vi "IEEE 754 Boolean_Array_to_SGL_LV2012_NI Verified.vi"(7 "array bool":bool[](array[boolean]), 10 "Tab Control":enum32{"SGL to Binary", "Binary to SGL"}(tab), 11 "Decimal Number":sgl=-101.101 format="%.12f") -> (3 "Decimal Number":sgl=-101.101 format="%.12f")   [LabVIEW 2015]
doc: "This VI shows how LabVIEW stores SGL floating-point numbers in memory in binary format. The 32-bit binary number is based on the following IEEE 754 format:\n\n1 bit for the SIGN\n8 bits for the EXPONENT\n23 bits for the MANTISSA\n\nThe formula for the conversion is the following:\n\nSGL = (-1)^SIGN * 1.MANTISSA * 2^(EXPONENT-127)\n\nYou can use this VI to convert SGL numbers to their binary storage equivalent, and vice versa."
panel:
  out "Decimal Exponent":sgl=6.0 format="%.2f"
  out "Decimal Mantissa":sgl=1.5797031 format="%.8f"
  out "Binary Mantissa":bool[](array[boolean])=[TRUE, FALSE, FALSE, TRUE, FALSE, TRUE, FALSE, FALSE, FALSE, TRUE, TRUE, FALSE, FALSE, TRUE, TRUE, TRUE, FALSE, TRUE, TRUE, FALSE, TRUE, TRUE, FALSE]
  out "Binary Exponent":bool[](array[boolean])=[TRUE, FALSE, FALSE, FALSE, FALSE, TRUE, FALSE, TRUE]
  out "Sign":bool=TRUE
  out "Sign":bool=TRUE
  out "Binary Exponent":bool[](array[boolean])=[TRUE, FALSE, FALSE, FALSE, FALSE, TRUE, FALSE, TRUE]
  out "Binary Mantissa":bool[](array[boolean])=[TRUE, FALSE, FALSE, TRUE, FALSE, TRUE, FALSE, FALSE, FALSE, TRUE, TRUE, FALSE, FALSE, TRUE, TRUE, TRUE, FALSE, TRUE, TRUE, FALSE, TRUE, TRUE, FALSE]
  out "Decimal Mantissa":sgl=1.5797031 format="%.8f"
  out "Decimal Exponent":i32=6
  # "Overview: This VI allows the conversion from and to IEEE 754 floating point\nRequirement: LabVIEW 2012 (or compatible)\nInstructions:\n1.  Choose a tab to convert from Binary to SGL or from SGL to binary\n2.  Enter your number in SGL or Binary\n3.  Run the VI"
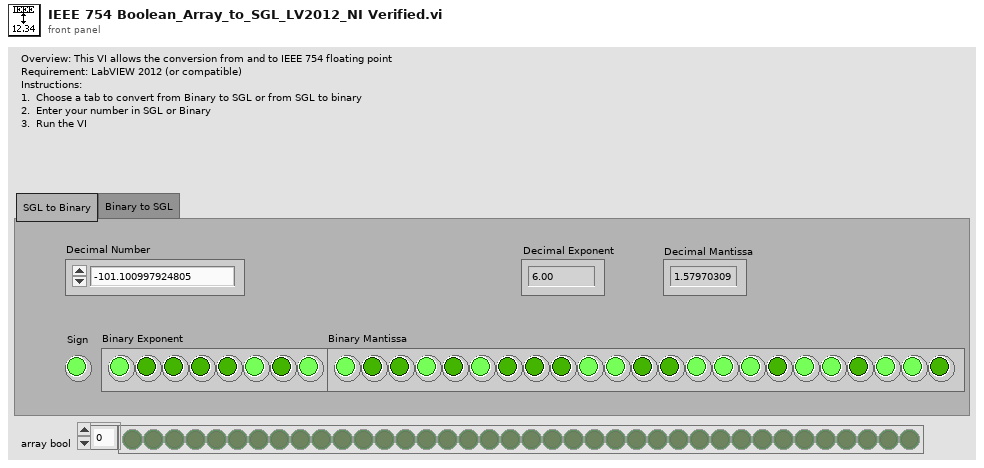
[diagram p1: front panel]
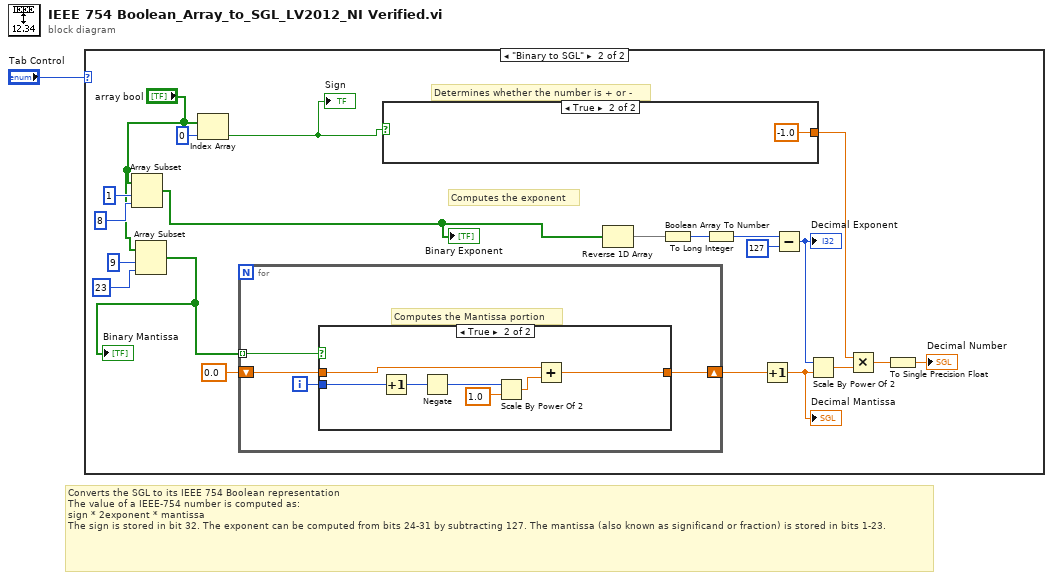
[diagram p0: block diagram]
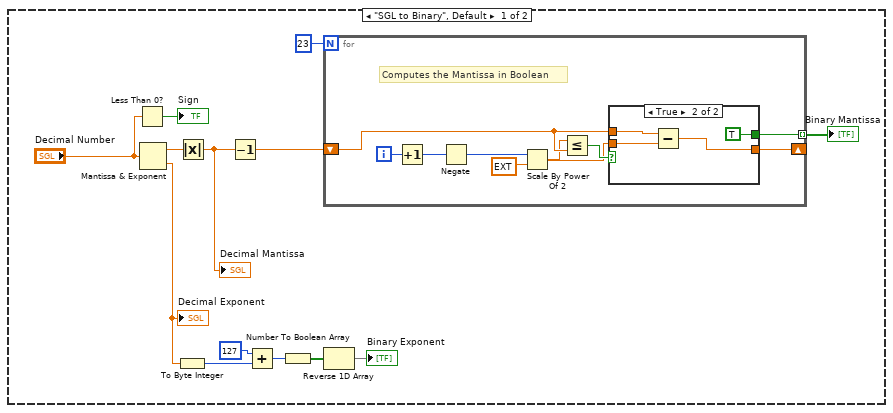
[diagram p2: hidden frame]
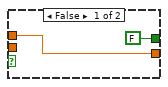
[diagram p3: hidden frame]
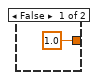
[diagram p4: hidden frame]
diagram:
  # "Converts the SGL to its IEEE 754 Boolean representation\nThe value of a IEEE-754 number is computed as:\nsign * 2exponent * mantissa\nThe sign is stored in bit 32. The exponent can be computed from bits 24-31 by subtracting 127. The mantissa (also known as significand or fraction) is stored in bits 1-23."
  n1 = case shown="\"Binary to SGL\"" "Tab Control" {
    frame "SGL to Binary", Default {
      n2 = Less Than 0?(x="Decimal Number") -> (x < 0?=→"Sign":bool)
      n3 = Mantissa & Exponent(0:"Decimal Number") -> (1:w4:sgl, 2:w8:sgl)
      "Decimal Exponent" <- w8
      n4 = To Byte Integer(number=w8) -> (8bit integer=w14:i8)
      n5 = Absolute Value(x=w4) -> (abs(x)=w5:sgl)
      "Decimal Mantissa" <- w5
      n6 = Decrement(x=w5) -> (x-1=w10:sgl)
      n7 = Add(x=i8 127, y=w14) -> (x+y=w13:i8)
      n8 = Number To Boolean Array(number=w13) -> (Boolean array=w12:bool[])
      n9 = for {
        N: 23 -> [_]
        shift-right: [w16] -> _
        shift-left: w10 -> [w18]
        tunnel: [w15] -> w3 mode=indexing
        i -> [w23]
        # "Computes the Mantissa in Boolean"
        n10 = Increment(x=w23) -> (x+1=w22:i32)
        n11 = Negate(x=w22) -> (-x=w21:i32)
        n12 = Scale By Power Of 2(n=w21, x=ext 1.0) -> (x*2^n=w17:ext)
        n13 = Less Or Equal?(x=w17, y=w18) -> (x <= y?=w19:bool)
        n14 = case shown="True" w19 {
          tunnel: w18 -> [w24 w29]
          tunnel: w17 -> [_ w26]
          tunnel: [w24 w28] -> w16
          tunnel: [FALSE TRUE] -> w15
          frame False {
          }
          frame True {
            n15 = Subtract(x=w29, y=w26) -> (x-y=w28:ext)
          }
        }
      }
      "Binary Mantissa" <- w3
      n16 = Reverse 1D Array(array=w12) -> (reversed array=→"Binary Exponent":bool[])
    }
    frame "Binary to SGL" {
      # "Computes the exponent"
      # "Determines whether the number is + or -"
      n17 = Array Subset(array="array bool", index=1, length=8 ("index")) -> (w31:bool[])
      "Binary Exponent" <- w31
      n18 = Array Subset(array="array bool", index=9, length=23 ("index")) -> (w30:bool[])
      "Binary Mantissa" <- w30
      n19 = Index Array(array="array bool", index=0) -> (element=w32:bool)
      "Sign" <- w32
      n20 = for {
        tunnel: w30 -> [w56] mode=indexing
        shift-right: [w53] -> w43
        shift-left: 0.0 -> [w54]
        i -> [w55]
        # "Computes the Mantissa portion"
        n21 = case shown="True" w56 {
          tunnel: w55 -> [_ w64]
          tunnel: w54 -> [w57 w60]
          tunnel: [w57 w58] -> w53
          frame False {
          }
          frame True {
            n22 = Increment(x=w64) -> (x+1=w63:i32)
            n23 = Negate(x=w63) -> (-x=w62:i32)
            n24 = Scale By Power Of 2(n=w62, x=1.0) -> (x*2^n=w59:dbl)
            n25 = Add(x=w60, y=w59) -> (x+y=w58:dbl)
          }
        }
      }
      n26 = case shown="True" w32 {
        tunnel: [1.0 -1.0] -> w48
        frame False {
        }
        frame True {
        }
      }
      n27 = Reverse 1D Array(array=w31) -> (reversed array=w46:bool[])
      n28 = Boolean Array To Number(Boolean array=w46) -> (number=w49:u32)
      n29 = To Long Integer(number=w49) -> (32bit integer=w50:i32)
      n30 = Increment(x=w43) -> (x+1=w41:dbl)
      "Decimal Mantissa" <- w41
      n31 = Subtract(x=w50, y=127) -> (x-y=w39:i32)
      "Decimal Exponent" <- w39
      n32 = Scale By Power Of 2(n=w39, x=w41) -> (x*2^n=w45:dbl)
      n33 = Multiply(x=w48, y=w45) -> (x*y=w47:dbl)
      n34 = To Single Precision Float(number=w47) -> (single precision float=→"Decimal Number":sgl)
    }
  }
